vi "SmartFileName.vi"(1 "Allow Replacement (False)":bool, 2 "preferred name":string, 3 "preferred path":path) -> (0 "Smart Path":path)   [LabVIEW 2016]
doc: "Creates unique filenames based on a preferred filepath."
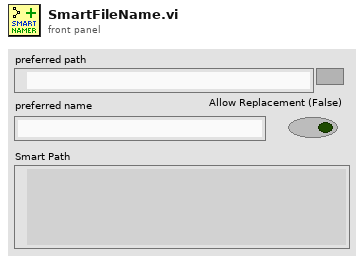
[diagram p1: front panel]
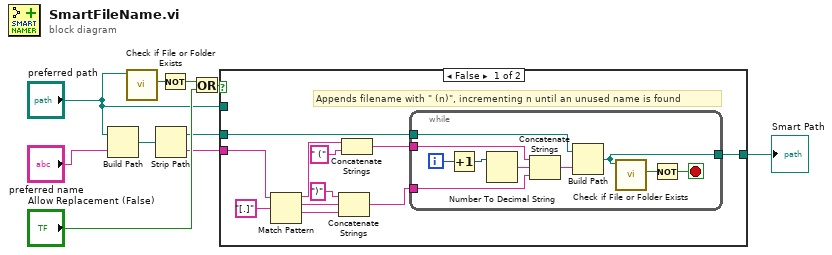
[diagram p0: block diagram]
diagram:
  n1 = Build Path(base path="preferred path", name or relative path="preferred name") -> (appended path=w2:path)
  n2 = call <vilib>:"Check if File or Folder Exists.vi"("path"="preferred path") -> ("file or folder exists?"=w10:bool)  [unwired: 8 in, 2 out]
  n3 = Strip Path(path=w2) -> (stripped path=w4:path, name=w3:string)
  n4 = Not(x=w10) -> (.not. x?=w6:bool)
  n5 = Or(x=w6, y="Allow Replacement (False)") -> (x .or. y?=w8:bool)
  n6 = case shown="False" w8 {
    tunnel: "preferred path" -> [_ w32]
    tunnel: w4 -> [w12 _]
    tunnel: w3 -> [w20 _]
    tunnel: [w11 w32] -> w9
    frame False {
      # "Appends filename with \" (n)\", incrementing n until an unused name is found"
      n7 = Match Pattern(string=w20, regular expression="[.]") -> (before substring=w14:string, match substring=w19:string, after substring=w18:string)  [unwired: 1 in, 1 out]
      n8 = Concatenate Strings(")", w19, w18) -> (w17:string)
      n9 = Concatenate Strings(w14, " (") -> (w13:string)
      n10 = while {
        tunnel: w17 -> [w28]
        tunnel: w13 -> [w29]
        tunnel: w12 -> [w26]
        tunnel: [w25] -> w11
        i -> [w31]
        stop <- w23 stop-if-true
        n11 = Increment(x=w31) -> (x+1=w22:i32)
        n12 = Number To Decimal String(number=w22) -> (decimal integer string=w30:string)  [unwired: 1 in]
        n13 = Concatenate Strings(w29, w30, w28) -> (w27:string)
        n14 = Build Path(base path=w26, name or relative path=w27) -> (appended path=w25:path)
        n15 = call <vilib>:"Check if File or Folder Exists.vi"("path"=w25) -> ("file or folder exists?"=w24:bool)  [unwired: 8 in, 2 out]
        n16 = Not(x=w24) -> (.not. x?=w23:bool)
      }
    }
    frame True {
    }
  }
  "Smart Path" <- w9
